vi "R2_Turn Pumps Off.vi"   [LabVIEW 2016]
uses:
  R2 DO Manual Control.ctl
  R2 Pump Manual Control.ctl
  R2 pH Manual Control.ctl
  R2Variables.lvlib
types:
  T1 = typedef "R2Variables.lvlib/R2 Pump Manual Control.ctl" = cluster{"Water Pump":bool, "Effluent Pump":bool, "Media Pump":bool, "Gas Pump":bool, "Air Release Valve":bool}
  T2 = typedef "R2 DO Manual Control.ctl" = cluster{"Air Valve":bool, "N2 Valve":bool}
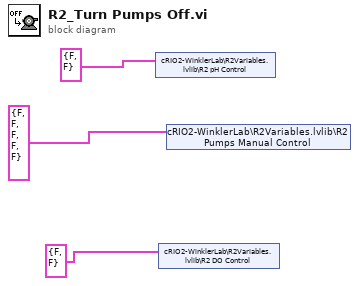
[diagram p0: block diagram]
diagram:
  n1 = shared-variable "cRIO2-WinklerLab\\R2Variables.lvlib\\R2 pH Control"(cluster{"Acid Pump":bool, "Base Pump":bool} {"Acid Pump"=FALSE, "Base Pump"=FALSE} ("Reactor 2 pH Control")) -> ()  [unwired: 1 in, 1 out]
  n2 = shared-variable "cRIO2-WinklerLab\\R2Variables.lvlib\\R2 DO Control"(T2 {"Air Valve"=FALSE, "N2 Valve"=FALSE} ("Reactor 2 DO Control")) -> ()  [unwired: 1 in, 1 out]
  n3 = shared-variable "cRIO2-WinklerLab\\R2Variables.lvlib\\R2 Pumps Manual Control"(T1 {"Water Pump"=FALSE, "Effluent Pump"=FALSE, "Media Pump"=FALSE, "Gas Pump"=FALSE, "Air Release Valve"=FALSE} ("Reactor 2 Pumps Manual Control")) -> ()  [unwired: 1 in, 1 out]
